vi "OSArchitecture.vi"(8 "error in (no error)":errorcluster) -> (0 "error out":errorcluster, 2 "32bit(T)/64bit(F)":bool)   [LabVIEW 2017]
panel:
  out "standard output":string
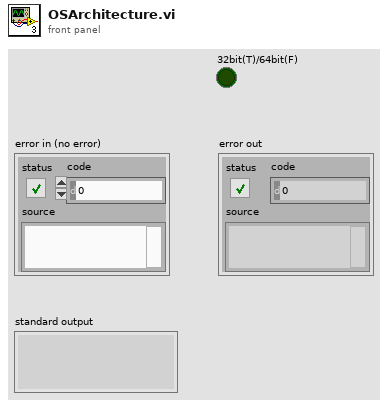
[diagram p1: front panel]
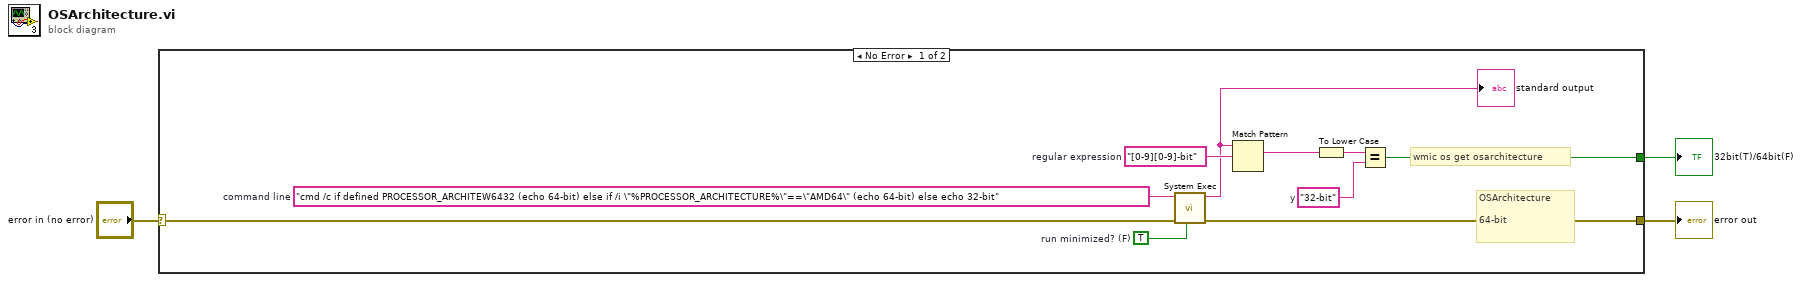
[diagram p0: block diagram]
diagram:
  n1 = case shown="No Error" "error in (no error)" {
    selector: "error in (no error)" -> [w4 w14]
    tunnel: [w7 w14] -> w2
    tunnel: [w5 _] -> w1
    frame No Error {
      w12 = TRUE  # run minimized? (F)
      w8 = "32-bit"  # y
      w11 = "[0-9][0-9]-bit"  # regular expression
      w13 = "cmd /c if defined PROCESSOR_ARCHITEW6432 (echo 64-bit) else if /i \"%PROCESSOR_ARCHITECTURE%\"==\"AMD64\" (echo 64-bit) else echo 32-bit"  # command line
      # "wmic os get osarchitecture"
      # "OSArchitecture  \n\n64-bit"
      n2 = call <vilib>:"System Exec.vi"("run minimized? (F)"=w12, "error in (no error)"=w4, "command line"=w13) -> ("error out"=w7:errorcluster, "standard output"=w6:string)  [unwired: 5 in, 2 out]
      "standard output" <- w6
      n3 = Match Pattern(string=w6, regular expression=w11) -> (match substring=w10:string)  [unwired: 1 in, 3 out]
      n4 = To Lower Case(string=w10) -> (all lower case string=w9:string)
      n5 = Equal?(x=w9, y=w8) -> (x = y?=w5:bool)
    }
    frame Error {
    }
  }
  "error out" <- w2
  "32bit(T)/64bit(F)" <- w1
